vi "MainApp.vi"() -> ()   [LabVIEW 2018]
uses:
  Typedefs/MainApp_SensorData_t.ctl
  Typedefs/MainApp_COMNotifier_t.ctl
  Typedefs/MainApp_DataQueue_t.ctl
  Typedefs/States_t.ctl
  <vilib>/Instr/_visa.llb/VISA Flush IO Buffer Mask.ctl
panel:
  in  "Tab Control":enum32{"Pomiar", "Obs³uga aplikacji", "Wykres"}(tab)
  out "Temperature values":dbl[][](array[numeric]) format="%.2f"
  out "Color box":u32[][](array[colorbox])
  out "Main loop":i32
  out "Task loop":i32
  out "Receiver loop":i32
  out "COM loop":i32
  out "For init":i32
  out "Amount of bytes received":u32
  in  "Stop application":bool
  in  "Cancel":bool
  in  "Virtual COM":refnum<visa-resource-name>
  in  "Close port button":bool
  in  "Open port button":bool
  out "Task loop error":errorcluster
  out "Main loop error":errorcluster
  out "Receiver loop error":errorcluster
  out "Receiving":bool
  out "COM port opened":bool
  out "Initialized":bool
  out "UI updated":bool
  out "COM port being opened":bool
  out "Trials of opening COM port":bool
  out "Sensor error occured":bool
  out "Temperature graph":T1(graph)
  out "Sensor Array":cluster{dbl, string}[](array[cluster])
  # "Aktualna temperatura w lodówce"
  # "Application state controls"
  # "Manual control of application"
  # "Debug counters"
  # "Application error reporters"
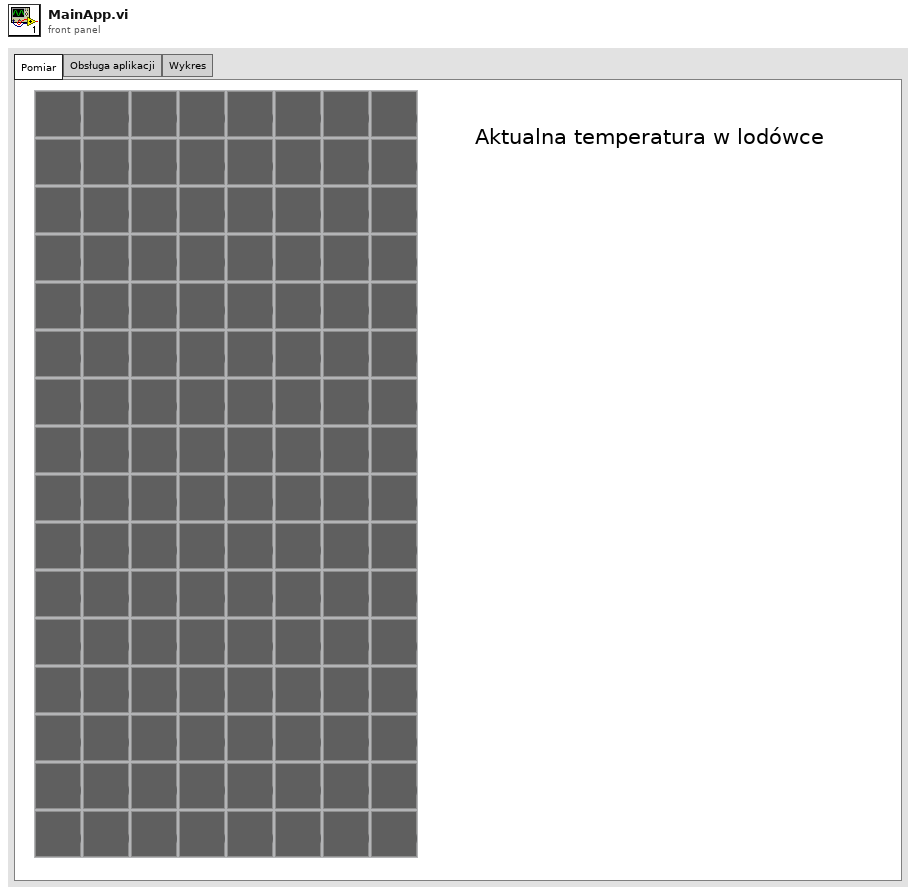
[diagram p1: front panel]
types:
  T1 = cluster{"[0]":dbl, "[1]":dbl, "[2]":dbl, "[3]":dbl, "[4]":dbl, "[5]":dbl, "[6]":dbl, "[7]":dbl, "[8]":dbl}
  T2 = typedef "MainApp_DataQueue_t.ctl" = cluster{"Next state":T3, "Received string":string}
  T3 = typedef "States_t.ctl" = enum16{"Initialize", "Wait", "Receive", "Process data", "Close port", "Open port", "Update UI", "End"}
  T4 = cluster{"Actual object height":dbl, "Actual object width":dbl}[]
  T5 = typedef "MainApp_COMNotifier_t.ctl" = cluster{"COM port":refnum<visa-resource-name>, "COM port opened":bool, "Stop operation":bool}
  T6 = typedef "MainApp_SensorData_t.ctl" = cluster{"Temperature value":dbl, "Sensor name":string, "Sensor enabled":bool, "Sensor number in receive list":i32, "Sensor location height":u8, "Sensor location width":u8, "Simulation weight":dbl[][], "Error occured":bool, "Ambient sensor":bool}[]
  T7 = cluster{"COM port":refnum<visa-resource-name>, "Received data":dbl[], "Received string":string, "COM port opened":bool, "Sensor data list":T6, "Sensor number":i32, "Simulation parameters [px]":cluster{"Object height":u8, "Object width":u8}, "Actual parameters [m]":cluster{"Object height":dbl, "Object width":dbl}, "Upper temperature bound":dbl, "Lower temperature bound":dbl}
  T8 = typedef "VISA Flush IO Buffer Mask.ctl" = u16
  T9 = cluster{"Temperature value":dbl, "Sensor name":string, "Sensor enabled":bool, "Sensor number in receive list":i32, "Sensor location height":u8, "Sensor location width":u8, "Simulation weight":dbl[][], "Error occured":bool, "Ambient sensor":bool}
  T10 = cluster{"Temperature value":dbl, "Sensor name":string}
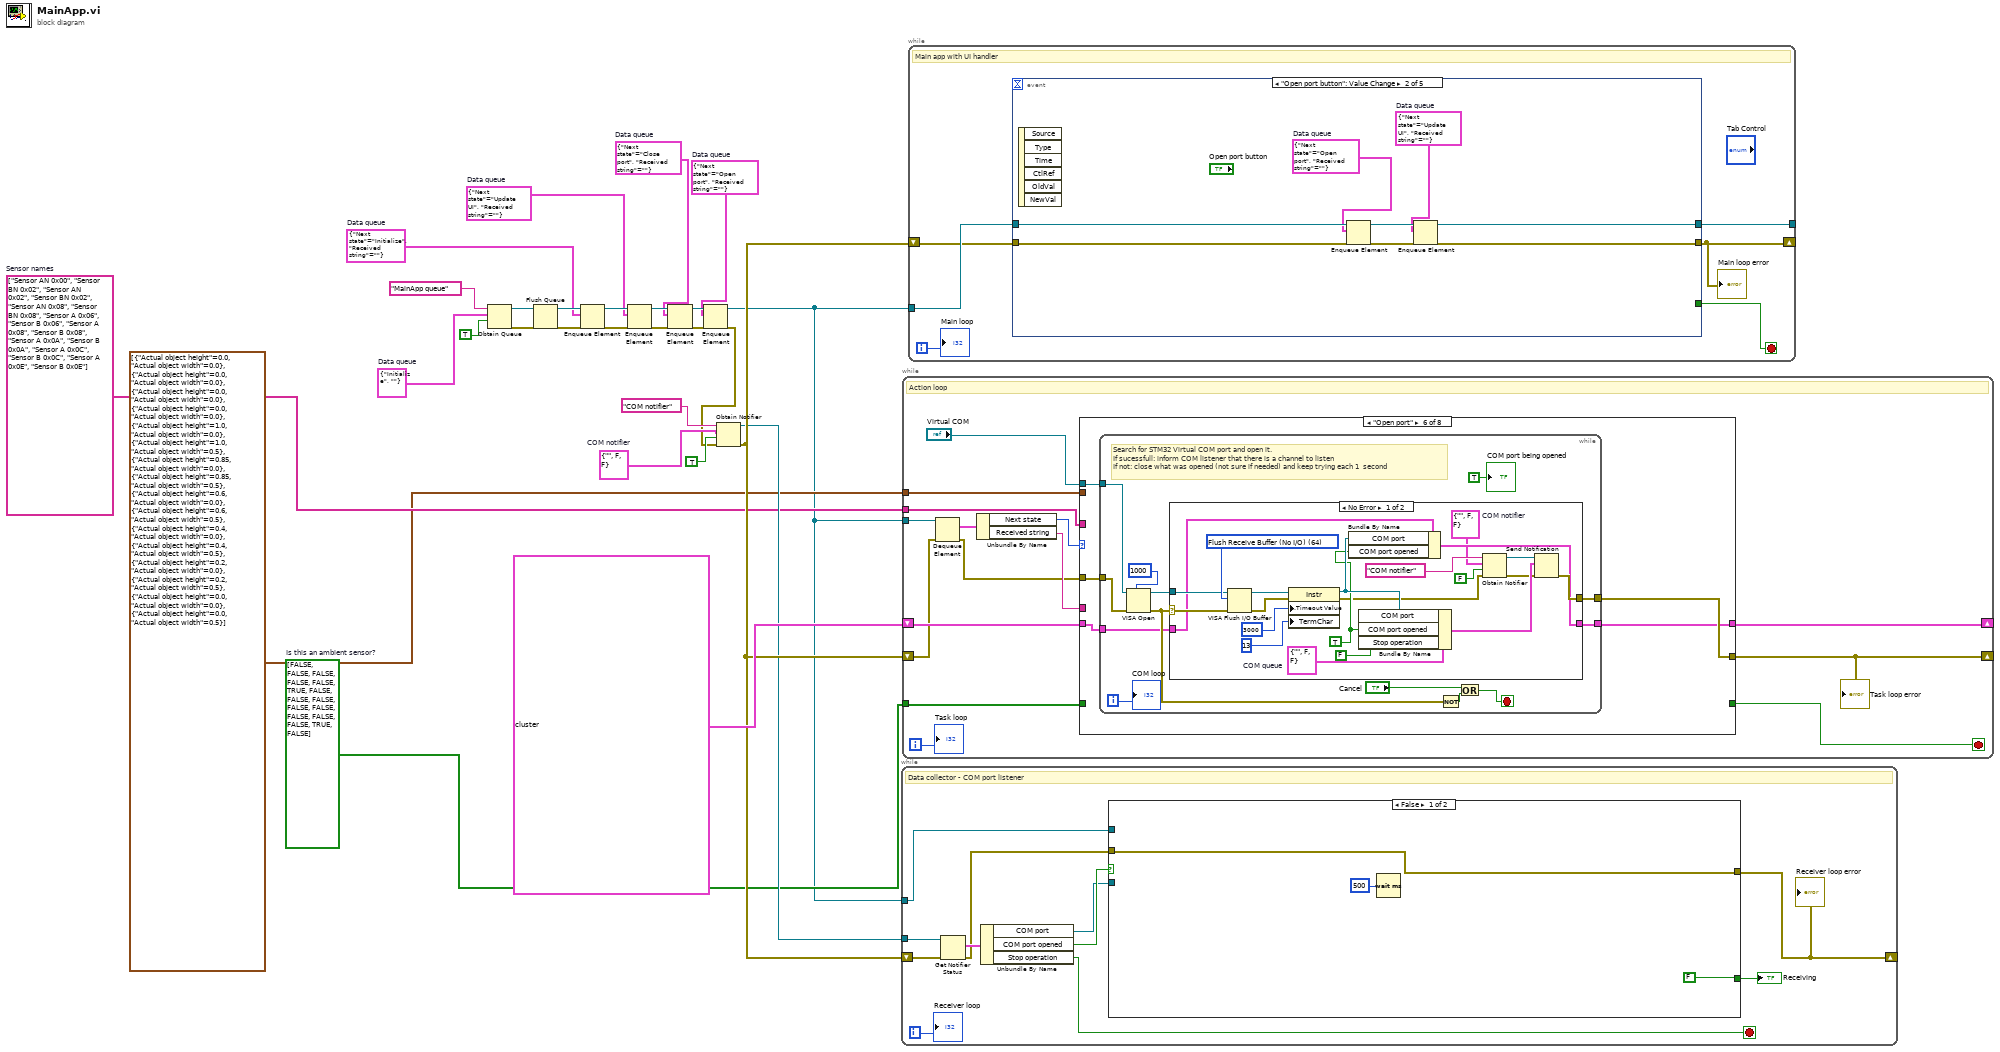
[diagram p0: block diagram]
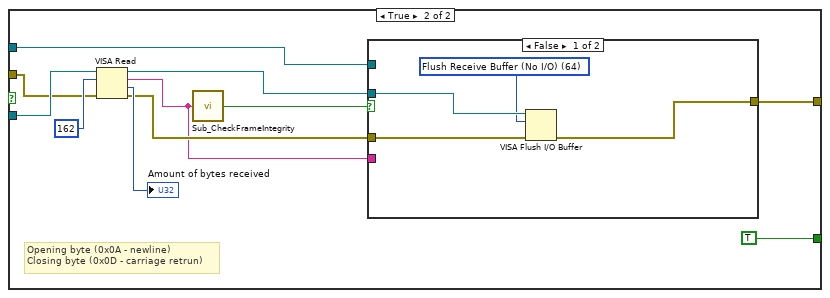
[diagram p2: hidden frame]
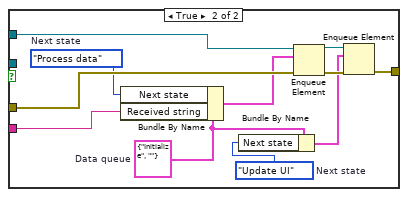
[diagram p3: hidden frame]
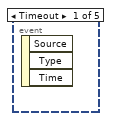
[diagram p4: hidden frame]
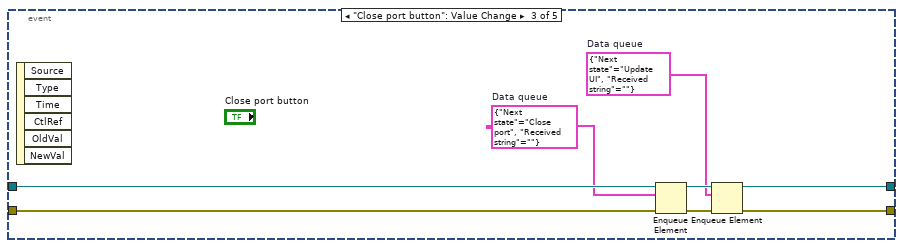
[diagram p5: hidden frame]
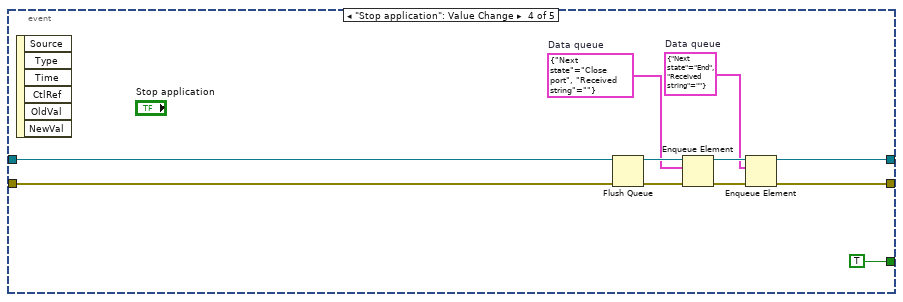
[diagram p6: hidden frame]
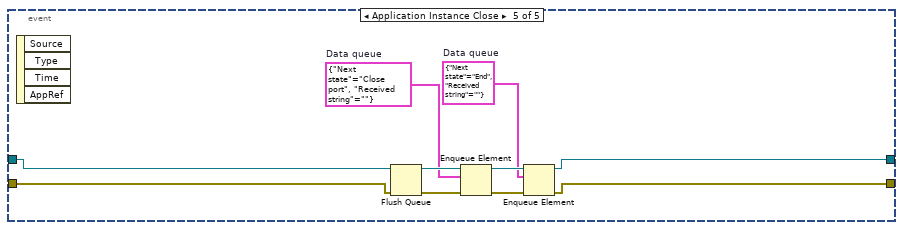
[diagram p7: hidden frame]
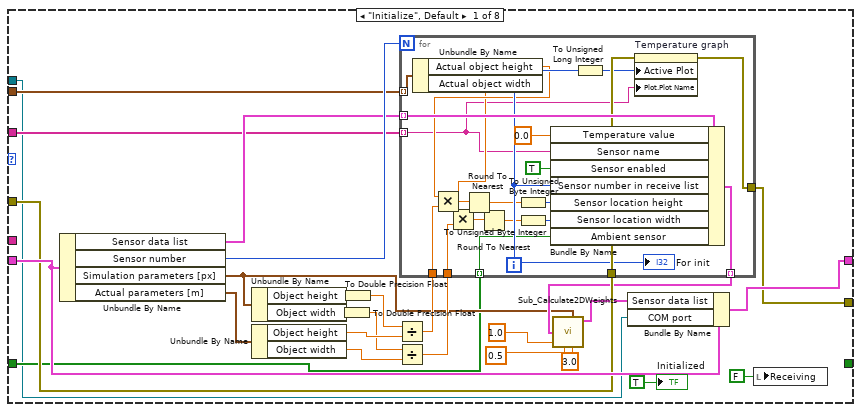
[diagram p8: hidden frame]
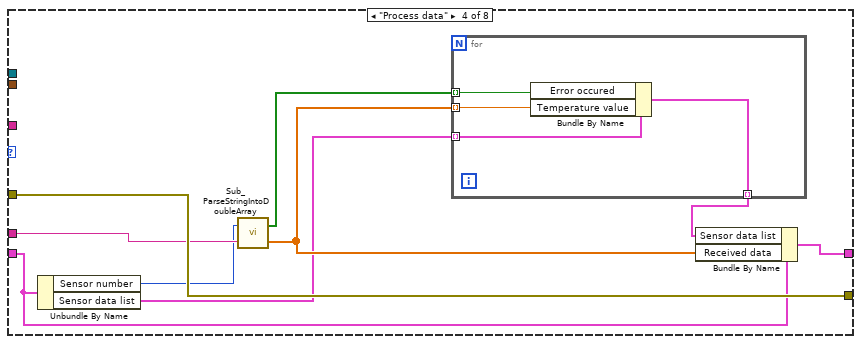
[diagram p11: hidden frame]
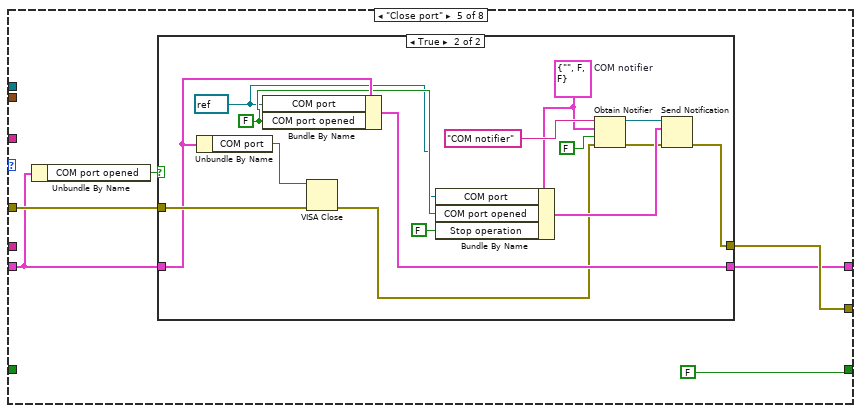
[diagram p12: hidden frame]
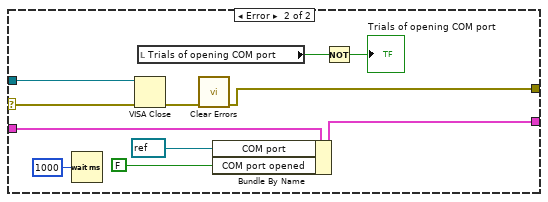
[diagram p14: hidden frame]
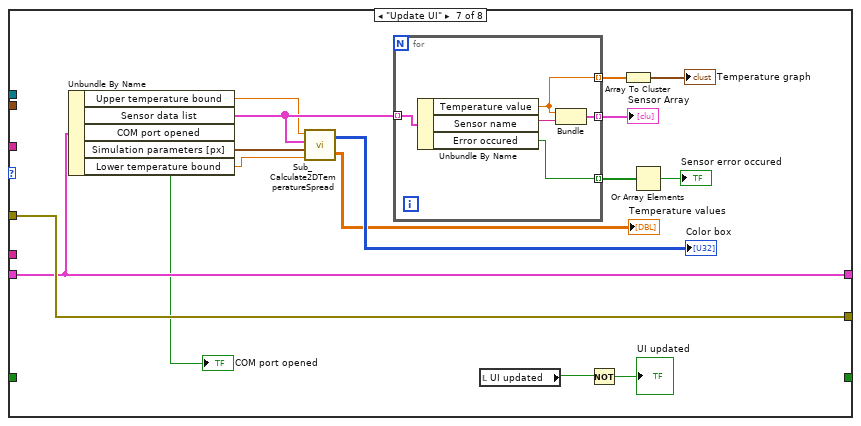
[diagram p15: hidden frame]
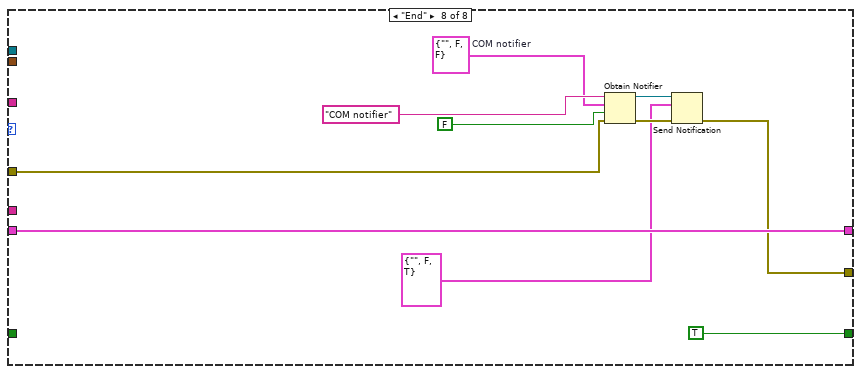
[diagram p16: hidden frame]
diagram:
  w1 = T2 {"Next state"=enum."Open port", "Received string"=""}  # Data queue
  w6 = T2 {"Next state"=enum."Close port", "Received string"=""}  # Data queue
  w9 = bool[] [FALSE, FALSE, FALSE, FALSE, FALSE, TRUE, FALSE, FALSE, FALSE, FALSE, FALSE, FALSE, FALSE, FALSE, TRUE, FALSE]  # Is this an ambient sensor?
  w11 = string[] ["Sensor AN 0x00", "Sensor BN 0x02", "Sensor AN 0x02", "Sensor BN 0x02", "Sensor AN 0x08", "Sensor BN 0x08", "Sensor A 0x06", "Sensor B 0x06", "Sensor A 0x08", "Sensor B 0x08", "Sensor A 0x0A", "Sensor B 0x0A", "Sensor A 0x0C", "Sensor B 0x0C", "Sensor A 0x0E", "Sensor B 0x0E"]  # Sensor names
  w13 = T2 {"Next state"=enum."Update UI", "Received string"=""}  # Data queue
  w14 = T2 {"Next state"=enum."Initialize", "Received string"=""}  # Data queue
  w20 = T2 {"Next state"=enum."Initialize", "Received string"=""}  # Data queue
  w22 = T5 {"COM port"="", "COM port opened"=FALSE, "Stop operation"=FALSE}  # COM notifier
  n1 = Obtain Queue(name (unnamed)="MainApp queue", element data type=w20, create if not found? (T)=TRUE) -> (queue out=w26:refnum<queue>, error out=w25:errorcluster)  [unwired: 2 in, 1 out]
  n2 = Flush Queue(queue=w26, error in (no error)=w25) -> (queue out=w19:refnum<queue>, error out=w18:errorcluster)  [unwired: 1 out]
  n3 = Enqueue Element(queue=w19, element=w14, error in (no error)=w18) -> (queue out=w17:refnum<queue>, error out=w16:errorcluster)  [unwired: 1 in, 1 out]
  n4 = Enqueue Element(queue=w17, element=w13, error in (no error)=w16) -> (queue out=w8:refnum<queue>, error out=w7:errorcluster)  [unwired: 1 in, 1 out]
  n5 = Enqueue Element(queue=w8, element=w6, error in (no error)=w7) -> (queue out=w2:refnum<queue>, error out=w5:errorcluster)  [unwired: 1 in, 1 out]
  n6 = Enqueue Element(queue=w2, element=w1, error in (no error)=w5) -> (queue out=w3:refnum<queue>, error out=w4:errorcluster)  [unwired: 1 in, 1 out]
  n7 = Obtain Notifier(name (unnamed)="COM notifier", notification data type=w22, create if not found? (T)=TRUE, error in (no error)=w4) -> (notifier out=w12:refnum<notifier>, error out=w15:errorcluster)  [unwired: 1 out]
  n8 = while {
    tunnel: w12 -> [w38]
    tunnel: w3 -> [w35]
    shift-right: [w29] -> _
    shift-left: w15 -> [w34]
    i -> [w31]
    stop <- w30 stop-if-true
    # "Data collector - COM port listener"
    n9 = Get Notifier Status(notifier=w38, error in (no error)=w34) -> (current notification=w37:T5, error out=w33:errorcluster)  [unwired: 3 out]
    n10 = Unbundle By Name(w37) -> ("COM port"=w36:refnum<visa-resource-name>, "COM port opened"=w39:bool, "Stop operation"=w30:bool)
    n11 = case shown="False" w39 {
      tunnel: w33 -> [w40 w50]
      tunnel: w36 -> [_ w51]
      tunnel: w35 -> [_ w46]
      tunnel: [FALSE TRUE] -> w32
      tunnel: [w40 w43] -> w29
      frame False {
        n12 = Wait (ms)(milliseconds to wait=u32 500) -> ()  [unwired: 1 out]
      }
      frame True {
        # "Opening byte (0x0A - newline)\nClosing byte (0x0D - carriage retrun)"
        n13 = VISA Read(VISA resource name=w51, byte count=u32 162, error in (no error)=w50) -> (VISA resource name out=w48:refnum<visa-resource-name>, read buffer=w45:string, return count=→"Amount of bytes received":u32, error out=w47:errorcluster)
        n14 = call "Sub_CheckFrameIntegrity.vi"("Received string"=w45) -> ("Is this valid frame?"=w49:bool)
        n15 = case shown="False" w49 {
          tunnel: w48 -> [w57 _]
          tunnel: w47 -> [w56 w64]
          tunnel: w46 -> [_ w68]
          tunnel: w45 -> [_ w67]
          tunnel: [w54 w58] -> w43
          frame False {
            w55 = T8 64 items=["Flush Receive Buffer"=16, "Write Transmit Buffer to Device"=32, "Flush Receive Buffer (No I/O)"=64, "Flush Transmit Buffer"=128] ("Mask")
            n16 = VISA Flush I/O Buffer(VISA resource name=w57, mask (16)=w55, error in (no error)=w56) -> (error out=w54:errorcluster)  [unwired: 1 out]
          }
          frame True {
            w59 = States_t."Update UI"  # Next state
            w60 = States_t."Process data"  # Next state
            w63 = T2 {"Next state"=enum."Initialize", "Received string"=""}  # Data queue
            n17 = Bundle By Name(cluster=w63, "Next state"=w60, "Received string"=w67) -> (w62:T2)
            n18 = Bundle By Name(cluster=w63, "Next state"=w59) -> (w61:T2)
            n19 = Enqueue Element(queue=w68, element=w62, error in (no error)=w64) -> (queue out=w66:refnum<queue>, error out=w65:errorcluster)  [unwired: 1 in, 1 out]
            n20 = Enqueue Element(queue=w66, element=w61, error in (no error)=w65) -> (error out=w58:errorcluster)  [unwired: 1 in, 2 out]
          }
        }
      }
    }
    "Receiving" <- w32
    "Receiver loop error" <- w29
    "Receiver loop" <- w31
  }
  n21 = while {
    shift-right: [w77] -> _
    shift-left: T7 {"COM port"="", "Received data"=[], "Received string"="", "COM port opened"=FALSE, "Sensor data list"=[{"Temperature value"=0.0, "Sensor name"="", "Sensor enabled"=FALSE, "Sensor number in receive list"=0, "Sensor location height"=0, "Sensor location width"=0, "Simulation weight"=[], "Error occured"=FALSE, "Ambient sensor"=FALSE}, {"Temperature value"=0.0, "Sensor name"="", "Sensor enabled"=TRUE, "Sensor number in receive list"=0, "Sensor location height"=0, "Sensor location width"=0, "Simulation weight"=[], "Error occured"=FALSE, "Ambient sensor"=FALSE}, {"Temperature value"=0.0, "Sensor name"="", "Sensor enabled"=TRUE, "Sensor number in receive list"=0, "Sensor location height"=0, "Sensor location width"=0, "Simulation weight"=[], "Error occured"=FALSE, "Ambient sensor"=FALSE}, {"Temperature value"=0.0, "Sensor name"="", "Sensor enabled"=TRUE, "Sensor number in receive list"=0, "Sensor location height"=0, "Sensor location width"=0, "Simulation weight"=[], "Error occured"=FALSE, "Ambient sensor"=FALSE}, {"Temperature value"=0.0, "Sensor name"="", "Sensor enabled"=TRUE, "Sensor number in receive list"=0, "Sensor location height"=0, "Sensor location width"=0, "Simulation weight"=[], "Error occured"=FALSE, "Ambient sensor"=FALSE}, {"Temperature value"=0.0, "Sensor name"="", "Sensor enabled"=TRUE, "Sensor number in receive list"=0, "Sensor location height"=0, "Sensor location width"=0, "Simulation weight"=[], "Error occured"=FALSE, "Ambient sensor"=FALSE}, {"Temperature value"=0.0, "Sensor name"="", "Sensor enabled"=TRUE, "Sensor number in receive list"=0, "Sensor location height"=0, "Sensor location width"=0, "Simulation weight"=[], "Error occured"=FALSE, "Ambient sensor"=FALSE}, {"Temperature value"=0.0, "Sensor name"="", "Sensor enabled"=TRUE, "Sensor number in receive list"=0, "Sensor location height"=0, "Sensor location width"=0, "Simulation weight"=[], "Error occured"=FALSE, "Ambient sensor"=FALSE}, {"Temperature value"=0.0, "Sensor name"="", "Sensor enabled"=TRUE, "Sensor number in receive list"=0, "Sensor location height"=0, "Sensor location width"=0, "Simulation weight"=[], "Error occured"=FALSE, "Ambient sensor"=FALSE}, {"Temperature value"=0.0, "Sensor name"="", "Sensor enabled"=TRUE, "Sensor number in receive list"=0, "Sensor location height"=0, "Sensor location width"=0, "Simulation weight"=[], "Error occured"=FALSE, "Ambient sensor"=FALSE}, {"Temperature value"=0.0, "Sensor name"="", "Sensor enabled"=TRUE, "Sensor number in receive list"=0, "Sensor location height"=0, "Sensor location width"=0, "Simulation weight"=[], "Error occured"=FALSE, "Ambient sensor"=FALSE}, {"Temperature value"=0.0, "Sensor name"="", "Sensor enabled"=TRUE, "Sensor number in receive list"=0, "Sensor location height"=0, "Sensor location width"=0, "Simulation weight"=[], "Error occured"=FALSE, "Ambient sensor"=FALSE}, {"Temperature value"=0.0, "Sensor name"="\n ", "Sensor enabled"=TRUE, "Sensor number in receive list"=0, "Sensor location height"=0, "Sensor location width"=0, "Simulation weight"=[], "Error occured"=FALSE, "Ambient sensor"=FALSE}, {"Temperature value"=0.0, "Sensor name"="", "Sensor enabled"=TRUE, "Sensor number in receive list"=0, "Sensor location height"=0, "Sensor location width"=0, "Simulation weight"=[], "Error occured"=FALSE, "Ambient sensor"=FALSE}, {"Temperature value"=0.0, "Sensor name"="", "Sensor enabled"=TRUE, "Sensor number in receive list"=0, "Sensor location height"=0, "Sensor location width"=0, "Simulation weight"=[], "Error occured"=FALSE, "Ambient sensor"=FALSE}, {"Temperature value"=0.0, "Sensor name"="", "Sensor enabled"=TRUE, "Sensor number in receive list"=0, "Sensor location height"=0, "Sensor location width"=0, "Simulation weight"=[], "Error occured"=FALSE, "Ambient sensor"=FALSE}], "Sensor number"=16, "Simulation parameters [px]"={"Object height"=16, "Object width"=8}, "Actual parameters [m]"={"Object height"=1.0, "Object width"=0.5}, "Upper temperature bound"=30.0, "Lower temperature bound"=20.0} -> [w83]
    shift-right: [w75] -> _
    shift-left: w15 -> [w81]
    tunnel: w3 -> [w82]
    tunnel: w11 -> [w72]
    tunnel: T4 [{"Actual object height"=0.0, "Actual object width"=0.0}, {"Actual object height"=0.0, "Actual object width"=0.0}, {"Actual object height"=0.0, "Actual object width"=0.0}, {"Actual object height"=0.0, "Actual object width"=0.0}, {"Actual object height"=1.0, "Actual object width"=0.0}, {"Actual object height"=1.0, "Actual object width"=0.5}, {"Actual object height"=0.85, "Actual object width"=0.0}, {"Actual object height"=0.85, "Actual object width"=0.5}, {"Actual object height"=0.6, "Actual object width"=0.0}, {"Actual object height"=0.6, "Actual object width"=0.5}, {"Actual object height"=0.4, "Actual object width"=0.0}, {"Actual object height"=0.4, "Actual object width"=0.5}, {"Actual object height"=0.2, "Actual object width"=0.0}, {"Actual object height"=0.2, "Actual object width"=0.5}, {"Actual object height"=0.0, "Actual object width"=0.0}, {"Actual object height"=0.0, "Actual object width"=0.5}] -> [w71]
    tunnel: w9 -> [w70]
    i -> [w74]
    stop <- w73 stop-if-true
    # "Action loop"
    n22 = Dequeue Element(queue=w82, error in (no error)=w81) -> (element=w80:T2, error out=w76:errorcluster)  [unwired: 1 in, 2 out]
    n23 = Unbundle By Name(w80) -> ("Next state"=w79:T3, "Received string"=w78:string)
    n24 = case shown="\"Open port\"" w79 {
      tunnel: w83 -> [w108 w133 w134 w140 w151 w174 w236 w252]
      tunnel: w76 -> [w105 w132 w135 w144 w154 w176 w237 w245]
      tunnel: [w106 w132 w135 w144 w153 w175 w237 w244] -> w75
      tunnel: w78 -> [_ _ _ w143 _ _ _ _]
      tunnel: [w107 w133 w134 w142 w152 w173 w236 w252] -> w77
      tunnel: [_ _ _ _ FALSE _ _ TRUE] -> w73
      tunnel: w72 -> [w87 _ _ _ _ _ _ _]
      tunnel: w71 -> [w86 _ _ _ _ _ _ _]
      tunnel: w70 -> [w85 _ _ _ _ _ _ _]
      tunnel: "Virtual COM" -> [w84 _ _ _ _ w172 _ _]
      frame "Initialize", Default {
        n25 = Unbundle By Name(w108) -> ("Sensor data list"=w109:T6, "Sensor number"=w110:i32, "Simulation parameters [px]"=w95:cluster{"Object height":u8, "Object width":u8}, "Actual parameters [m]"=w102:cluster{"Object height":dbl, "Object width":dbl})
        n26 = Unbundle By Name(w95) -> ("Object height"=w101:u8, "Object width"=w100:u8)
        n27 = Unbundle By Name(w102) -> ("Object height"=w90:dbl, "Object width"=w88:dbl)
        n28 = To Double Precision Float(number=w100) -> (double precision float=w89:dbl)
        n29 = To Double Precision Float(number=w101) -> (double precision float=w91:dbl)
        n30 = Divide(x=w91, y=w90) -> (x/y=w99:dbl)
        n31 = Divide(x=w89, y=w88) -> (x/y=w98:dbl)
        n32 = for {
          N: w110 -> [_]
          tunnel: w109 -> [w131] mode=indexing
          tunnel: [w128] -> w97 mode=indexing
          tunnel: w105 -> [w127]
          tunnel: [w126] -> w106
          tunnel: w99 -> [w122]
          tunnel: w98 -> [w115]
          tunnel: w87 -> [w114] mode=indexing
          tunnel: w86 -> [w113] mode=indexing
          tunnel: w85 -> [w112] mode=indexing
          i -> [w125]
          n33 = Unbundle By Name(w113) -> ("Actual object height"=w123:dbl, "Actual object width"=w116:dbl)
          n34 = Multiply(x=w123, y=w122) -> (x*y=w124:dbl)
          n35 = Multiply(x=w116, y=w115) -> (x*y=w118:dbl)
          n36 = Round To Nearest(number=w124) -> (nearest integer value=w121:dbl)
          n37 = Round To Nearest(number=w118) -> (nearest integer value=w119:dbl)
          n38 = To Unsigned Byte Integer(number=w121) -> (unsigned 8bit integer=w120:u8)
          n39 = To Unsigned Byte Integer(number=w119) -> (unsigned 8bit integer=w117:u8)
          n40 = Bundle By Name(cluster=w131, "Temperature value"=0.0, "Sensor name"=w114, "Sensor enabled"=TRUE, "Sensor number in receive list"=w125, "Sensor location height"=w120, "Sensor location width"=w117, "Ambient sensor"=w112) -> (w128:T9)
          n41 = To Unsigned Long Integer(number=w125) -> (unsigned 32bit integer=w111:u32)
          n42 = property on="Temperature graph" class="WFChart (strict)"(error in=w127, "Active Plot"=w111, "Plot.Plot Name"=w114) -> (error out=w126:errorcluster)  [unwired: 1 in, 1 out]
          "For init" <- w125
        }
        n43 = call "Sub_Calculate2DWeights.vi"("Sensor data list"=w97, "Height scaling"=1.0, "Width scaling"=0.5, "Simulation parameters"=w95, "Standard deviation"=3.0) -> ("Sensor information output"=w96:T6)  [unwired: 5 in]
        n44 = Bundle By Name(cluster=w108, "Sensor data list"=w96, "COM port"=w84) -> (w107:T7)
        n45 = local write "Receiving"(FALSE ("Receiving")) -> ()
        "Initialized" <- TRUE
      }
      frame "Wait" {
      }
      frame "Receive" {
      }
      frame "Process data" {
        n46 = Unbundle By Name(w140) -> ("Sensor number"=w139:i32, "Sensor data list"=w138:T6)
        n47 = call "Sub_ParseStringIntoDoubleArray.vi"("Received string"=w143, "Number of active sensors"=w139) -> ("Output data"=w141:dbl[], "Error array"=w136:bool[])
        n48 = for {
          tunnel: w141 -> [w147] mode=indexing
          tunnel: w138 -> [w148] mode=indexing
          tunnel: [w146] -> w137 mode=indexing
          tunnel: w136 -> [w145] mode=indexing
          n49 = Bundle By Name(cluster=w148, "Error occured"=w145, "Temperature value"=w147) -> (w146:T9)
        }
        n50 = Bundle By Name(cluster=w140, "Sensor data list"=w137, "Received data"=w141) -> (w142:T7)
      }
      frame "Close port" {
        n51 = Unbundle By Name(w151) -> ("COM port opened"=w150:bool)
        n52 = case shown="True" w150 {
          tunnel: w154 -> [w156 w171]
          tunnel: [w156 w157] -> w153
          tunnel: w151 -> [w155 w169]
          tunnel: [w155 w168] -> w152
          frame False {
          }
          frame True {
            w159 = T5 {"COM port"="", "COM port opened"=FALSE, "Stop operation"=FALSE}  # COM notifier
            w161 = FALSE ("COM port opened")
            w160 = refnum<visa-resource-name> refnum ("COM port")
            n53 = Unbundle By Name(w169) -> ("COM port"=w170:refnum<visa-resource-name>)
            n54 = Bundle By Name(cluster=w169, "COM port"=w160, "COM port opened"=w161) -> (w168:T7)
            n55 = VISA Close(VISA resource name=w170, error in (no error)=w171) -> (error out=w158:errorcluster)
            n56 = Bundle By Name(cluster=w159, "COM port"=w160, "COM port opened"=w161, "Stop operation"=FALSE) -> (w167:T5)
            n57 = Obtain Notifier(name (unnamed)="COM notifier", notification data type=w159, create if not found? (T)=FALSE, error in (no error)=w158) -> (notifier out=w164:refnum<notifier>, error out=w163:errorcluster)  [unwired: 1 out]
            n58 = Send Notification(notification=w167, notifier=w164, error in (no error)=w163) -> (error out=w157:errorcluster)  [unwired: 1 out]
          }
        }
      }
      frame "Open port" {
        n59 = while {
          tunnel: w176 -> [w187]
          tunnel: [w185] -> w175
          tunnel: w174 -> [w184]
          tunnel: [w183] -> w173
          tunnel: w172 -> [w180]
          i -> [w181]
          stop <- w179 stop-if-true
          # "Search for STM32 Virtual COM port and open it. \nIf sucessfull: inform COM listener that there is a channel to listen\nIf not: close what was opened (not sure if needed) and keep trying each 1  second"
          n60 = VISA Open(timeout (0)=u32 1000 ("VISA Open timeout (0)"), error in (no error)=w187, VISA resource name=w180) -> (VISA resource name=w189:refnum<visa-resource-name>, error out=w186:errorcluster)  [unwired: 2 in]
          n61 = case shown="No Error" w186 {
            selector: w186 -> [w210 w219]
            tunnel: w189 -> [w206 w218]
            tunnel: [w201 w213] -> w185
            tunnel: w184 -> [w199 w217]
            tunnel: [w200 w216] -> w183
            frame No Error {
              w195 = T5 {"COM port"="", "COM port opened"=FALSE, "Stop operation"=FALSE}  # COM notifier
              w197 = TRUE ("COM port opened")
              w203 = T5 {"COM port"="", "COM port opened"=FALSE, "Stop operation"=FALSE}  # COM queue
              w209 = T8 64 items=["Flush Receive Buffer"=16, "Write Transmit Buffer to Device"=32, "Flush Receive Buffer (No I/O)"=64, "Flush Transmit Buffer"=128] ("Mask")
              n62 = VISA Flush I/O Buffer(VISA resource name=w206, mask (16)=w209, error in (no error)=w210) -> (VISA resource name out=w205:refnum<visa-resource-name>, error out=w204:errorcluster)
              n63 = property class="Instr"(reference=w205, error in=w204, "General Settings:Timeout Value"=u32 3000, "TermChar"=u8 13 ("Message Based Settings:Termination Character")) -> (reference out=w198:refnum<visa-resource-name>, error out=w191:errorcluster)
              n64 = Bundle By Name(cluster=w199, "COM port"=w198, "COM port opened"=w197) -> (w200:T7)
              n65 = Bundle By Name(cluster=w203, "COM port"=w198, "COM port opened"=w197, "Stop operation"=FALSE) -> (w202:T5)
              n66 = Obtain Notifier(name (unnamed)="COM notifier", notification data type=w195, create if not found? (T)=FALSE, error in (no error)=w191) -> (notifier out=w193:refnum<notifier>, error out=w192:errorcluster)  [unwired: 1 out]
              n67 = Send Notification(notification=w202, notifier=w193, error in (no error)=w192) -> (error out=w201:errorcluster)  [unwired: 1 out]
            }
            frame Error {
              n68 = Wait (ms)(milliseconds to wait=u32 1000) -> ()  [unwired: 1 out]
              n69 = VISA Close(VISA resource name=w218, error in (no error)=w219) -> (error out=w220:errorcluster)
              n70 = local read "Trials of opening COM port"() -> (w211:bool)
              n71 = call <vilib>:"Clear Errors.vi"("error in (no error)"=w220) -> ("error out"=w213:errorcluster)  [unwired: 5 in, 1 out]
              n72 = Bundle By Name(cluster=w217, "COM port"=refnum<visa-resource-name> refnum, "COM port opened"=FALSE) -> (w216:T7)
              n73 = Not(x=w211) -> (.not. x?=→"Trials of opening COM port":bool)
            }
          }
          n74 = Not(x=w186) -> (.not. x?=w178:bool)
          n75 = Or(x="Cancel", y=w178) -> (x .or. y?=w179:bool)
          "COM loop" <- w181
          "COM port being opened" <- TRUE
        }
      }
      frame "Update UI" {
        n76 = Unbundle By Name(w236) -> ("Upper temperature bound"=w229:dbl, "Sensor data list"=w230:T6, "COM port opened"=→"COM port opened":bool, "Simulation parameters [px]"=w231:cluster{"Object height":u8, "Object width":u8}, "Lower temperature bound"=w228:dbl)
        n77 = call "Sub_Calculate2DTemperatureSpread.vi"("Upper temperature bound"=w229, "Sensor data list"=w230, "Simulation parameters"=w231, "Lower temperature bound"=w228) -> ("Output color boxes"=→"Color box":u32[][], "Temperature values"=→"Temperature values":dbl[][])  [unwired: 1 in]
        n78 = for {
          tunnel: w230 -> [w242] mode=indexing
          tunnel: [w240] -> w232 mode=indexing
          tunnel: [w239] -> w234 mode=indexing
          tunnel: [w238] -> w227 mode=indexing
          n79 = Unbundle By Name(w242) -> ("Temperature value"=w239:dbl, "Sensor name"=w241:string, "Error occured"=w238:bool)
          n80 = Bundle("Temperature value"=w239, "Sensor name"=w241) -> (w240:T10)  [unwired: 1 in]
        }
        "Sensor Array" <- w232
        n81 = local read "UI updated"() -> (w225:bool)
        n82 = Not(x=w225) -> (.not. x?=→"UI updated":bool)
        n83 = Array To Cluster(array=w234) -> (cluster=→"Temperature graph":T1)
        n84 = Or Array Elements(Boolean array=w227) -> (logical OR=→"Sensor error occured":bool)
      }
      frame "End" {
        w249 = T5 {"COM port"="", "COM port opened"=FALSE, "Stop operation"=FALSE}  # COM notifier
        n85 = Obtain Notifier(name (unnamed)="COM notifier", notification data type=w249, create if not found? (T)=FALSE, error in (no error)=w245) -> (notifier out=w247:refnum<notifier>, error out=w246:errorcluster)  [unwired: 1 out]
        n86 = Send Notification(notification=T5 {"COM port"="", "COM port opened"=FALSE, "Stop operation"=TRUE}, notifier=w247, error in (no error)=w246) -> (error out=w244:errorcluster)  [unwired: 1 out]
      }
    }
    "Task loop error" <- w75
    "Task loop" <- w74
  }
  n87 = while {
    tunnel: w3 -> [w258]
    tunnel: [w256] -> _
    shift-right: [w255] -> _
    shift-left: w15 -> [w257]
    i -> [w254]
    stop <- w253 stop-if-true
    # "Main app with UI handler"
    n88 = event shown="[1] \"Open port button\": Value Change" {
      selector: _ -> [_ _ _ _ _]
      dyn-events: _ -> [_ _ _ _ _]
      timeout: _ -> [_ _ _ _ _]
      tunnel: w258 -> [_ w266 w274 w281 w286]
      tunnel: w257 -> [_ w265 w273 w280 w287]
      tunnel: [_ w260 w268 w277 w289] -> w256
      tunnel: [_ w259 w267 w283 w288] -> w255
      tunnel: [_ _ _ TRUE _] -> w253
      event Timeout {
        n89 = event-data() -> ()  [unwired: 1 in, 3 out]
      }
      event "Open port button": Value Change {
        w261 = T2 {"Next state"=enum."Update UI", "Received string"=""}  # Data queue
        w264 = T2 {"Next state"=enum."Open port", "Received string"=""}  # Data queue
        n90 = event-data() -> ()  [unwired: 1 in, 6 out]
        n91 = Enqueue Element(queue=w266, element=w264, error in (no error)=w265) -> (queue out=w262:refnum<queue>, error out=w263:errorcluster)  [unwired: 1 in, 1 out]
        n92 = Enqueue Element(queue=w262, element=w261, error in (no error)=w263) -> (queue out=w260:refnum<queue>, error out=w259:errorcluster)  [unwired: 1 in, 1 out]
      }
      event "Close port button": Value Change {
        w269 = T2 {"Next state"=enum."Update UI", "Received string"=""}  # Data queue
        w272 = T2 {"Next state"=enum."Close port", "Received string"=""}  # Data queue
        n93 = event-data() -> ()  [unwired: 1 in, 6 out]
        n94 = Enqueue Element(queue=w274, element=w272, error in (no error)=w273) -> (queue out=w271:refnum<queue>, error out=w270:errorcluster)  [unwired: 1 in, 1 out]
        n95 = Enqueue Element(queue=w271, element=w269, error in (no error)=w270) -> (queue out=w268:refnum<queue>, error out=w267:errorcluster)  [unwired: 1 in, 1 out]
      }
      event "Stop application": Value Change {
        w275 = T2 {"Next state"=enum."Close port", "Received string"=""}  # Data queue
        w276 = T2 {"Next state"=enum."End", "Received string"=""}  # Data queue
        n96 = event-data() -> ()  [unwired: 1 in, 6 out]
        n97 = Flush Queue(queue=w281, error in (no error)=w280) -> (queue out=w279:refnum<queue>, error out=w282:errorcluster)  [unwired: 1 out]
        n98 = Enqueue Element(queue=w279, element=w275, error in (no error)=w282) -> (queue out=w278:refnum<queue>, error out=w284:errorcluster)  [unwired: 1 in, 1 out]
        n99 = Enqueue Element(queue=w278, element=w276, error in (no error)=w284) -> (queue out=w277:refnum<queue>, error out=w283:errorcluster)  [unwired: 1 in, 1 out]
      }
      event Application Instance Close {
        w290 = T2 {"Next state"=enum."Close port", "Received string"=""}  # Data queue
        w291 = T2 {"Next state"=enum."End", "Received string"=""}  # Data queue
        n100 = event-data() -> ()  [unwired: 1 in, 4 out]
        n101 = Flush Queue(queue=w286, error in (no error)=w287) -> (queue out=w293:refnum<queue>, error out=w294:errorcluster)  [unwired: 1 out]
        n102 = Enqueue Element(queue=w293, element=w290, error in (no error)=w294) -> (queue out=w292:refnum<queue>, error out=w295:errorcluster)  [unwired: 1 in, 1 out]
        n103 = Enqueue Element(queue=w292, element=w291, error in (no error)=w295) -> (queue out=w289:refnum<queue>, error out=w288:errorcluster)  [unwired: 1 in, 1 out]
      }
    }
    "Main loop error" <- w255
    "Main loop" <- w254
  }
